vi "RSZVB Define Pulse Train Segments.vi"(5 "Pulse Train Active":i32[](array[numeric]), 6 "Stop Time":dbl[](array[numeric]) format="%^.3e", 7 "Start Time":dbl[](array[numeric]) format="%^.3e", 8 "error in (no error)":errorcluster {"code" format="%.0x"}, 10 "Channel (1)":i32=1, 11 "VISA session":refnum<visa-resource-name>) -> (0 "error out":errorcluster {"code" format="%.0x"}, 3 "dup VISA session":refnum<visa-resource-name>)   [LabVIEW 2011]
doc: "This VI adds and enables/disables an arbitrary number of pulse train segments. Each segment consists of a single pulse of definite width and position which may be active or inactive.\n\nNote(s):\n\n(1) This VI is available only with option R&S ZVA-K27.\n\nRemote-control command(s):\n[SENSe<Ch>:]PULSe:GENerator<gen_no>:TRAin:DATA <Active>, <Start High>, <Stop High>{, <Active>, <Start High>, <Stop High>}"
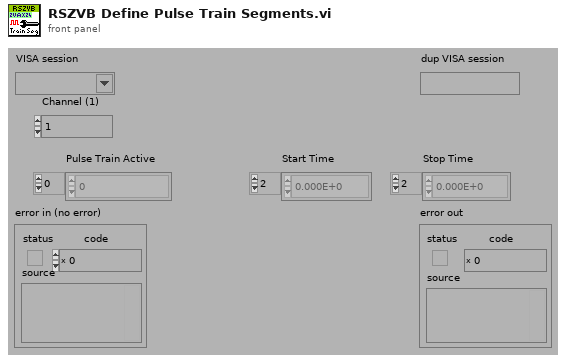
[diagram p1: front panel]
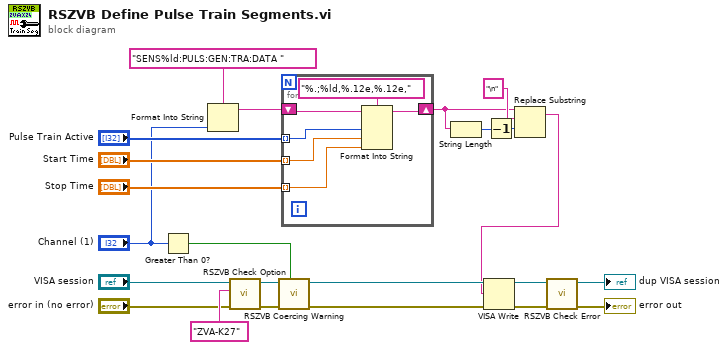
[diagram p0: block diagram]
diagram:
  n1 = Greater Than 0?(x="Channel (1)") -> (x > 0?=w16:bool)
  n2 = Format Into String(format string="SENS%ld:PULS:GEN:TRA:DATA ", "Channel (1)") -> (resulting string=w8:string)  [unwired: 2 in, 1 out]
  n3 = call "RSZVB Check Option.vi"("error in (no error)"="error in (no error)", "Options"="ZVA-K27", "VISA session"="VISA session") -> ("error out"=w18:errorcluster, "dup VISA session"=w17:refnum<visa-resource-name>)  [unwired: 7 in]
  n4 = call "RSZVB Coercing Warning.vi"("In Range?"=w16, "error in (no error)"=w18, "VISA session"=w17) -> ("error out"=w22:errorcluster, "dup VISA session"=w23:refnum<visa-resource-name>)  [unwired: 7 in]
  n5 = for {
    tunnel: "Pulse Train Active" -> [w27] mode=indexing
    tunnel: "Start Time" -> [w26] mode=indexing
    tunnel: "Stop Time" -> [w25] mode=indexing
    shift-right: [w24] -> w6
    shift-left: w8 -> [w28]
    n6 = Format Into String(format string="%.;%ld,%.12e,%.12e,", initial string=w28, w27, w26, w25) -> (resulting string=w24:string)  [unwired: 1 in, 1 out]
  }
  n7 = String Length(string=w6) -> (length=w5:i32)
  n8 = Decrement(x=w5) -> (x-1=w3:i32)
  n9 = Replace Substring(3:w3, 4:"\n" ("substring (\"\")"), 5:w6) -> (1:w4:string)  [unwired: 1 in, 1 out]
  n10 = VISA Write(VISA resource name=w23, write buffer=w4, error in (no error)=w22) -> (VISA resource name out=w20:refnum<visa-resource-name>, error out=w21:errorcluster)  [unwired: 1 out]
  n11 = call "RSZVB Check Error.vi"("error in (no error)"=w21, "VISA session"=w20) -> ("error out"=→"error out":errorcluster, "dup VISA session"=→"dup VISA session":refnum<visa-resource-name>)  [unwired: 8 in]
